vi "Export File - Rx XML.vi"(6 "RootNode":refnum<k24>, 7 "Rx Packets":T1 {"Rx Packet Data"."targetPriority" min=-2 max=16 step=1; "Rx Packet Data"."targetProcessor" min=-2 max=16 step=1; "Rx Packet Data"."Endianness" items=["big-endian"=0, "little-endian"=2]}, 8 "error in (no error)":errorcluster, 11 "XmlDocument in":refnum<k24>) -> (0 "error out":errorcluster, 3 "XmlDocument out":refnum<k24>)   [LabVIEW 2019, in "UDP-Custom-Device System Explorer.lvlib"]
uses:
  UDP-Custom-Device System Explorer.lvlib
  System.Xml
  Types/XML - New/ImpExp - Rx Packets Data.ctl
  <vilib>/NI VeriStand/Custom Device API/Custom Device Item Info.ctl
  Types/XML - New/ImpExp - Rx Packet Data.ctl
  Shared/Types/Shared - Channel Data Type.ctl
  Shared/Types/Shared - Buffered.PacketInfo.ctl
  Shared/Types/Shared - Pointer Encoding.ctl
  Shared/Types/Shared - Receive Buffer Options.ctl
  Shared/Types/Shared - Transmit Buffer Options.ctl
  Shared/Types/Shared - New Data Options.ctl
  Shared/Types/Shared - Thread Management.ctl
  Types/XML - New/ImpExp - Packet Headers.ctl
  <vilib>/NI VeriStand/Custom Device API/Custom Device API.lvlib
  Shared/UDP-Custom-Device Shared.lvlib
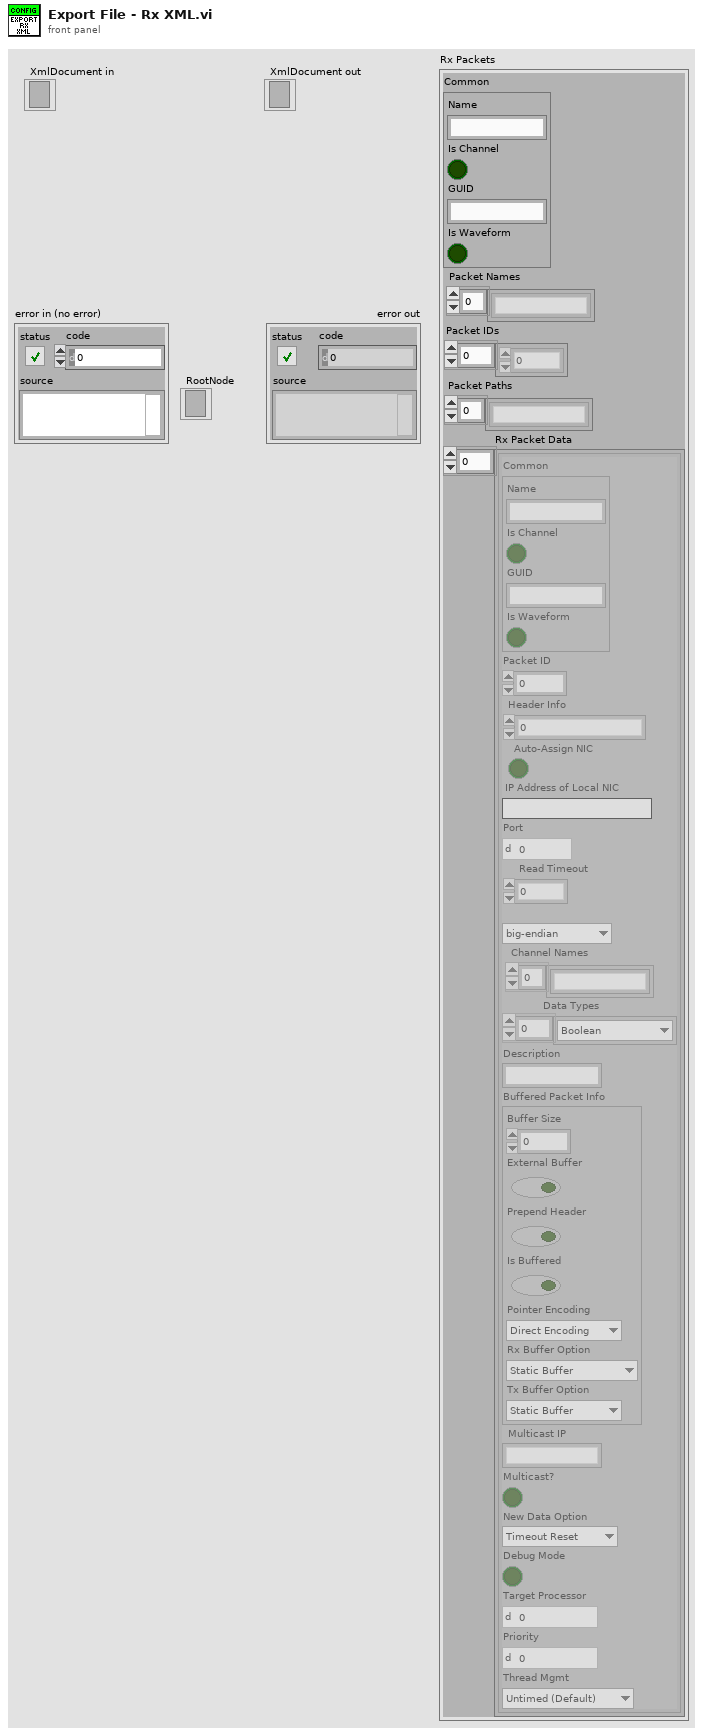
[diagram p1: front panel]
types:
  T1 = typedef "UDP-Custom-Device System Explorer.lvlib/ImpExp - Rx Packets Data.ctl" = cluster{"Common":T2, "Packet Names":string[], "Packet IDs":i32[], "Packet Paths":string[], "Rx Packet Data":T3[]}
  T2 = typedef "Custom Device API.lvlib/Custom Device Item Info.ctl" = cluster{"Name":string, "Is Channel":bool, "GUID":string, "Is Waveform":bool}
  T3 = typedef "UDP-Custom-Device System Explorer.lvlib/ImpExp - Rx Packet Data.ctl" = cluster{"Common":T2, "Packet ID":i32, "Header Info":u32, "Auto-Assign NIC":bool, "IP Address of Local NIC":string, "Port":u16, "Read Timeout":i32, "Endianness":u16, "Channel Names":string[], "Data Types":T4[], "Description":string, "Buffered Packet Info":T5, "Multicast IP":string, "Multicast?":bool, "New Data Option":T9, "Debug Mode":bool, "targetProcessor":i8, "targetPriority":i16, "Thread Mgmt":T10}
  T4 = typedef "UDP-Custom-Device Shared.lvlib/Shared - Channel Data Type.ctl" = enum16{"Boolean", "Single", "Double", "I8", "I16", "I32", "I64", "U8", "U16", "U32", "U64"}
  T5 = typedef "UDP-Custom-Device Shared.lvlib/Shared - Buffered.PacketInfo.ctl" = cluster{"Buffer Size":i32, "External Buffer":bool, "Prepend Header":bool, "Is Buffered":bool, "Pointer Encoding":T6, "Rx Buffer Option":T7, "Tx Buffer Option":T8}
  T6 = typedef "UDP-Custom-Device Shared.lvlib/Shared - Pointer Encoding.ctl" = enum16{"Direct Encoding", "Conversion Encoding"}
  T7 = typedef "UDP-Custom-Device Shared.lvlib/Shared - Receive Buffer Options.ctl" = enum16{"Static Buffer", "Circular Buffer", "Circular Buffer + Size", "Internal Cache", "Internal Cache + Size", "Ping Pong", "Ping Pong + Size"}
  T8 = typedef "UDP-Custom-Device Shared.lvlib/Shared - Transmit Buffer Options.ctl" = enum16{"Static Buffer", "FIFO Buffer", "FIFO Buffer + Port"}
  T9 = typedef "UDP-Custom-Device Shared.lvlib/Shared - New Data Options.ctl" = enum16{"Timeout Reset", "Counter"}
  T10 = typedef "UDP-Custom-Device Shared.lvlib/Shared - Thread Management.ctl" = enum16{"Untimed (Default)", "Timed (High Priority)"}
  T11 = typedef "UDP-Custom-Device System Explorer.lvlib/ImpExp - Packet Headers.ctl" = cluster{"Packet Name":string, "Packet ID":string, "Packet Path":string}
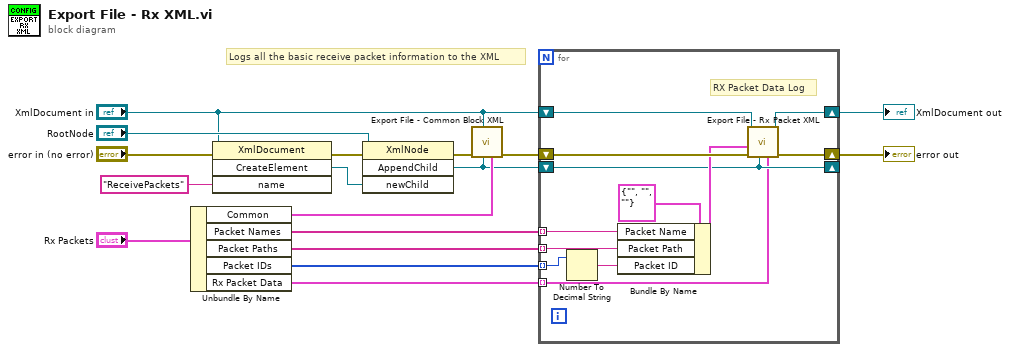
[diagram p0: block diagram]
diagram:
  # "Logs all the basic receive packet information to the XML"
  n1 = Unbundle By Name("Rx Packets") -> ("Common"=w12:T2, "Packet Names"=w6:string[], "Packet Paths"=w1:string[], "Packet IDs"=w5:i32[], "Rx Packet Data"=w3:T3[])
  n2 = invoke class="XmlDocument" method="CreateElement"(reference="XmlDocument in", error in="error in (no error)", "name"="ReceivePackets" ("Tag Name")) -> (error out=w16:errorcluster, "CreateElement"=w15:refnum<k24>)  [unwired: 1 in, 2 out]
  n3 = invoke class="XmlNode" method="AppendChild"(reference="RootNode", error in=w16, "newChild"=w15) -> (error out=w17:errorcluster, "AppendChild"=w10:refnum<k24>)  [unwired: 1 in, 2 out]
  n4 = call "Export File - Common Block XML.vi"("Common"=w12, "RootNode in"=w10, "XmlDocument in"="XmlDocument in", "error in (no error)"=w17) -> ("error out"=w9:errorcluster)  [unwired: 7 in]
  n5 = for {
    shift-right: [w26] -> w7
    shift-left: w9 -> [w27]
    shift-right: [w28] -> w8
    shift-left: "XmlDocument in" -> [w29]
    tunnel: w6 -> [w24] mode=indexing
    tunnel: w5 -> [w23] mode=indexing
    shift-right: [w19] -> _
    shift-left: w10 -> [w19]
    tunnel: w3 -> [w18] mode=indexing
    tunnel: w1 -> [w21] mode=indexing
    # "RX Packet Data Log"
    n6 = Number To Decimal String(number=w23) -> (decimal integer string=w22:string)  [unwired: 1 in]
    n7 = Bundle By Name(cluster=T11 {"Packet Name"="", "Packet ID"="", "Packet Path"=""} ("Rx Packet XML Data"), "Packet Name"=w24, "Packet Path"=w21, "Packet ID"=w22) -> (w20:T11)
    n8 = call "Export File - Rx Packet XML.vi"("Rx Packet"=w18, "RootNode"=w19, "error in (no error)"=w27, "Rx Packet Header Data"=w20, "XmlDocument in"=w29) -> ("error out"=w26:errorcluster, "XmlDocument out"=w28:refnum<k24>)  [unwired: 5 in]
  }
  "error out" <- w7
  "XmlDocument out" <- w8
